vi "Custom wrapped 10 bit counter.vi"(9 "increment or decrement (decrement)":bool, 10 "max value":fxp<+,10,10>, 11 "value":fxp<+,10,10>) -> (2 "wrapped":bool, 3 "new value":fxp<+,10,10>)   [LabVIEW 2017, in "Engine Simulation Toolkit System Explorer.lvlib"]
uses:
  Engine Simulation Toolkit System Explorer.lvlib
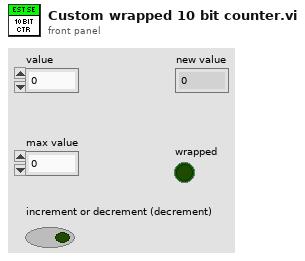
[diagram p1: front panel]
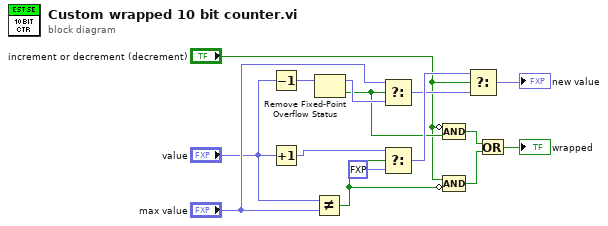
[diagram p0: block diagram]
diagram:
  n1 = Decrement(x="value") -> (x-1=w15:fxp<+,10,10>)
  n2 = Increment(x="value") -> (x+1=w14:fxp<+,10,10>)
  n3 = Not Equal?(x="value", y="max value") -> (x != y?=w5:bool)
  n4 = Remove Fixed-Point Overflow Status(3:w15) -> (0:w7:bool, 1:w11:fxp<+,10,10>)
  n5 = Select(t="max value", s=w7, f=w11) -> (s? t:f=w8:fxp<+,10,10>)
  n6 = Select(t=w14, s=w5, f=fxp<+,10,10> 0.0) -> (s? t:f=w9:fxp<+,10,10>)
  n7 = Compound Arithmetic op=AND(invert "increment or decrement (decrement)", w7) -> (w4:bool)
  n8 = Compound Arithmetic op=AND("increment or decrement (decrement)", invert w5) -> (w3:bool)
  n9 = Select(t=w9, s="increment or decrement (decrement)", f=w8) -> (s? t:f=→"new value":fxp<+,10,10>)
  n10 = Or(x=w4, y=w3) -> (x .or. y?=→"wrapped":bool)
